vi "OBJ_parse_read_gear_data_response.vi"(8 "error_in":errorcluster, 11 "recordset_in":variant) -> (0 "error_out":errorcluster, 2 "Perform test?":bool)   [LabVIEW 2019]
uses:
  FGV/tristate_indicator_OBJ_test/FGV_tristate_indicator_OBJ_test.ctl
  FGV/test_button/FGV_OBJ_test_button.ctl
  <vilib>/addons/database/_DB Variant To Data/Database Variant To Data.xnode
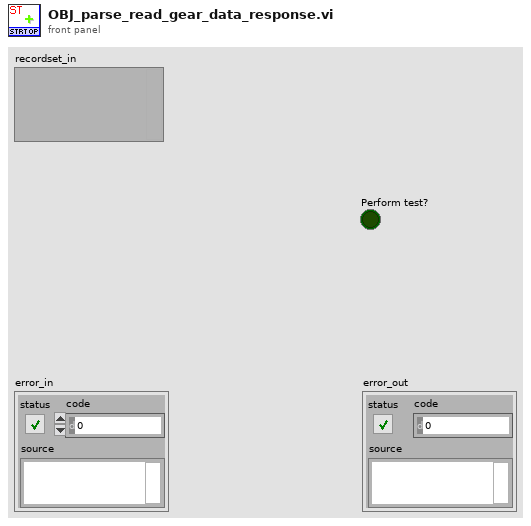
[diagram p1: front panel]
types:
  T1 = typedef "FGV_OBJ_test_button.ctl" = enum16{"initialize", "set_new_login", "set_message", "enable", "disable", "disable_gray", "translate"}
  T2 = typedef "FGV_tristate_indicator_OBJ_test.ctl" = enum16{"initialize", "ready", "pending", "OK", "NOK", "part_NOK", "routing_NOK", "repeat_NOK", "timeout", "translate", "error"}
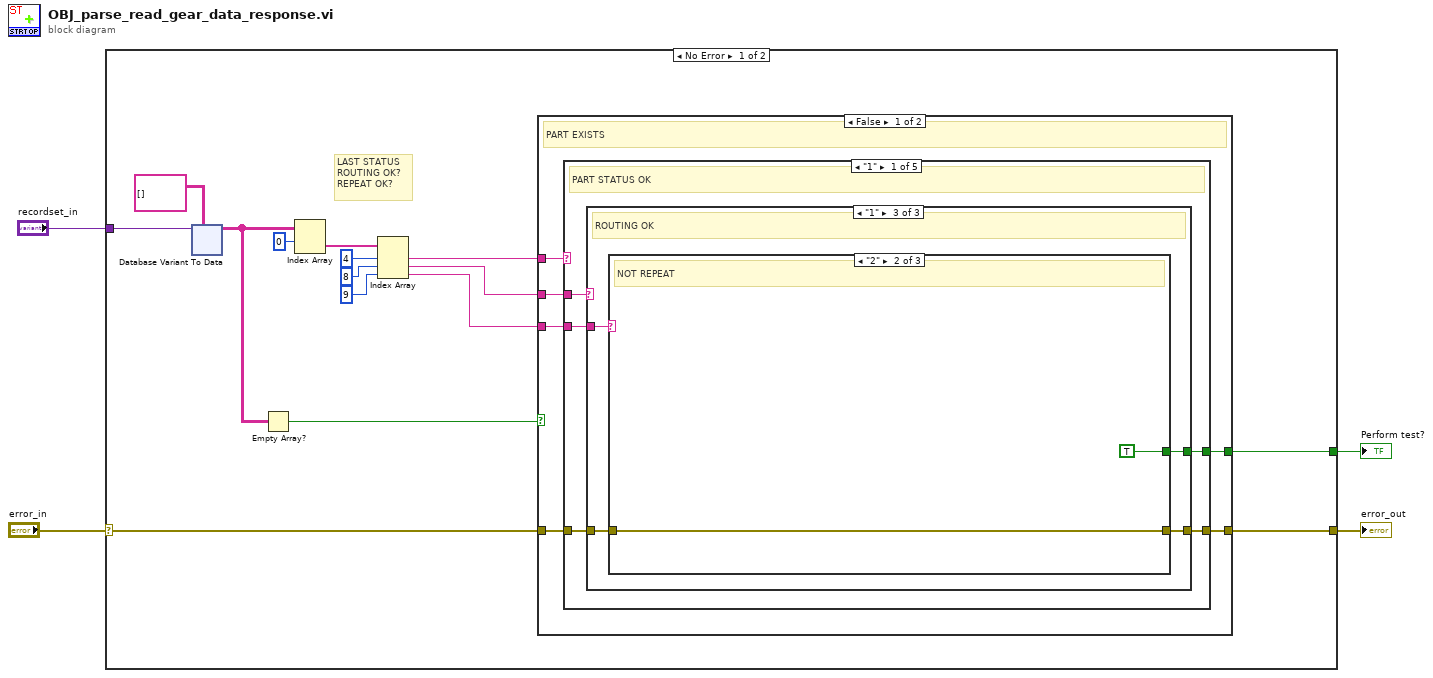
[diagram p0: block diagram]
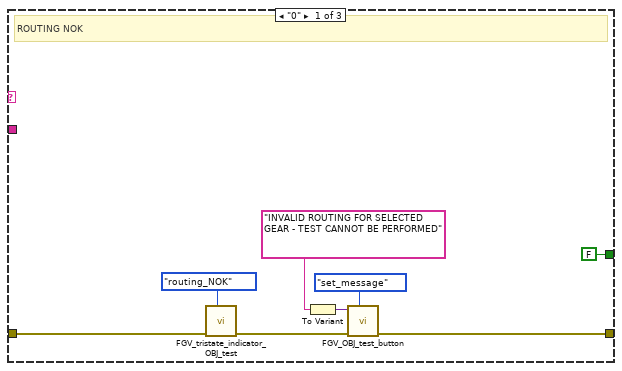
[diagram p2: hidden frame]
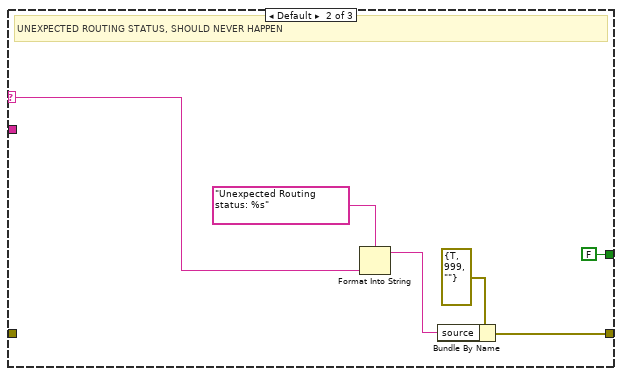
[diagram p3: hidden frame]
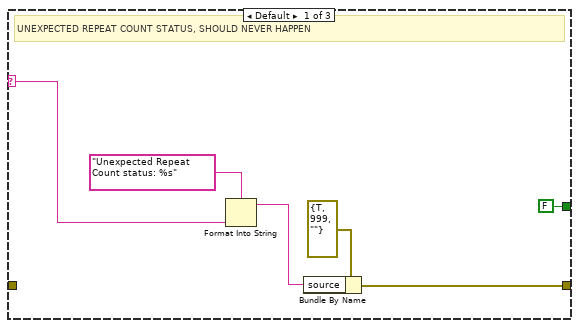
[diagram p4: hidden frame]
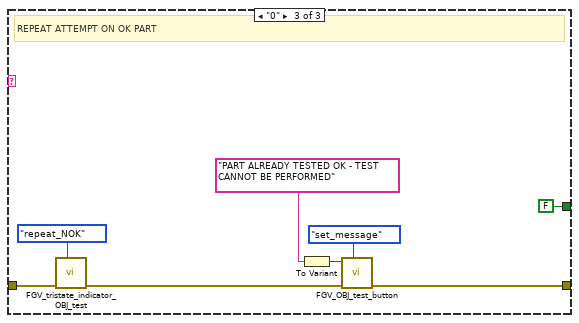
[diagram p5: hidden frame]
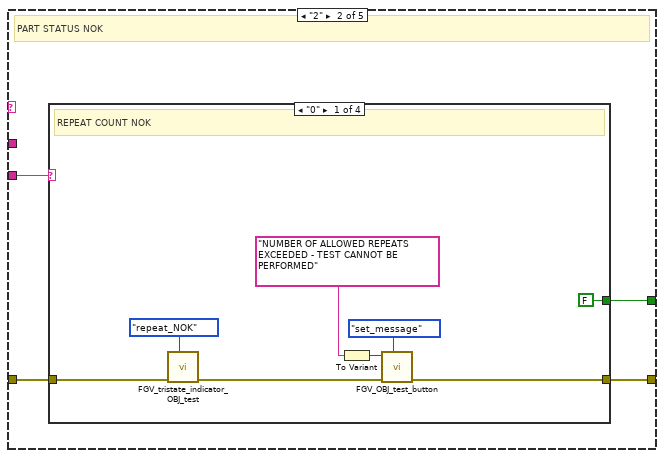
[diagram p6: hidden frame]
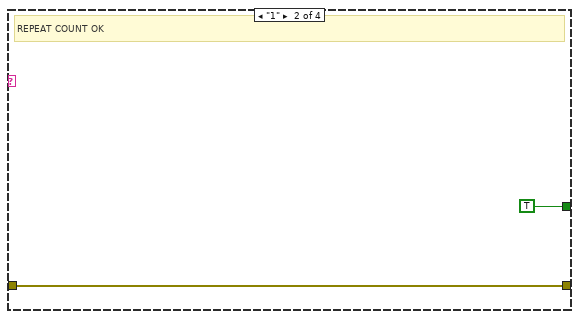
[diagram p7: hidden frame]
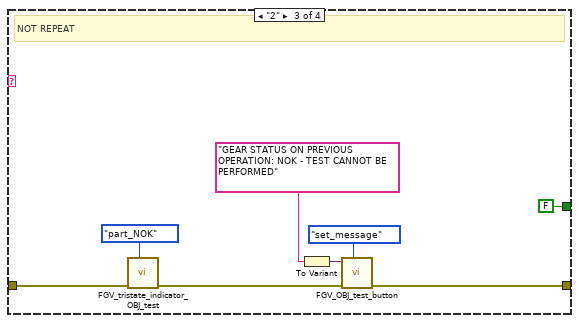
[diagram p8: hidden frame]
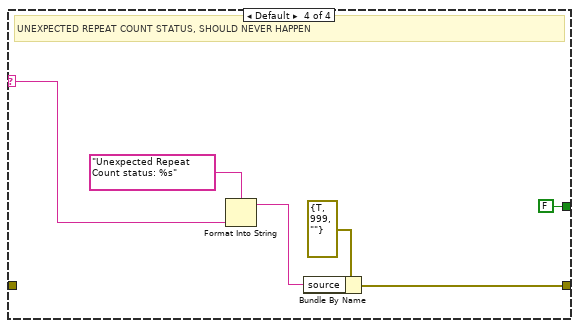
[diagram p9: hidden frame]
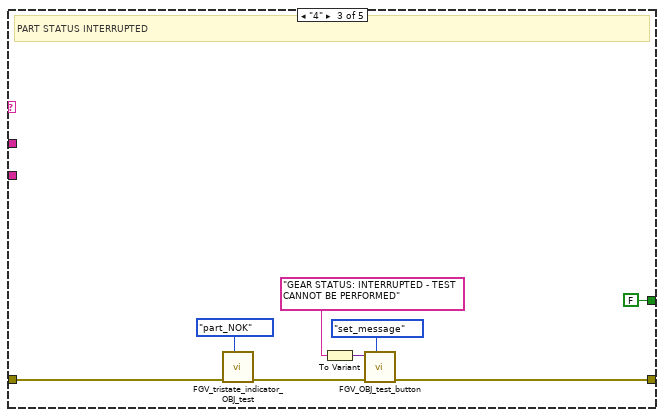
[diagram p10: hidden frame]
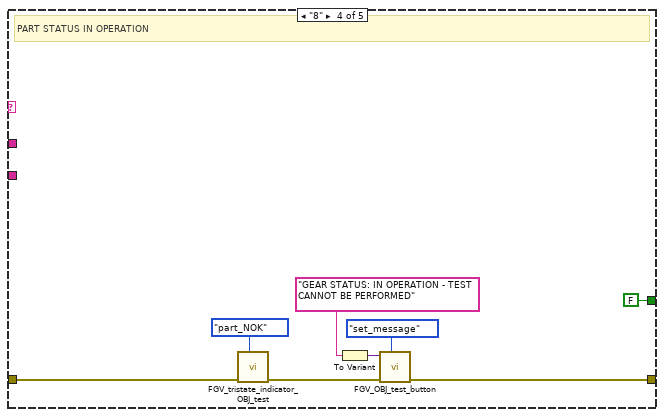
[diagram p11: hidden frame]
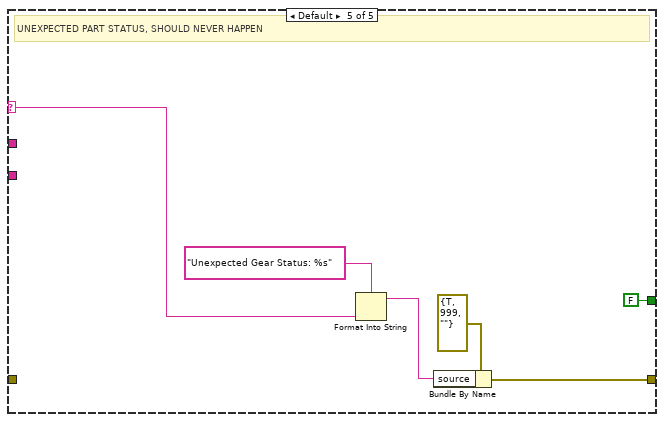
[diagram p12: hidden frame]
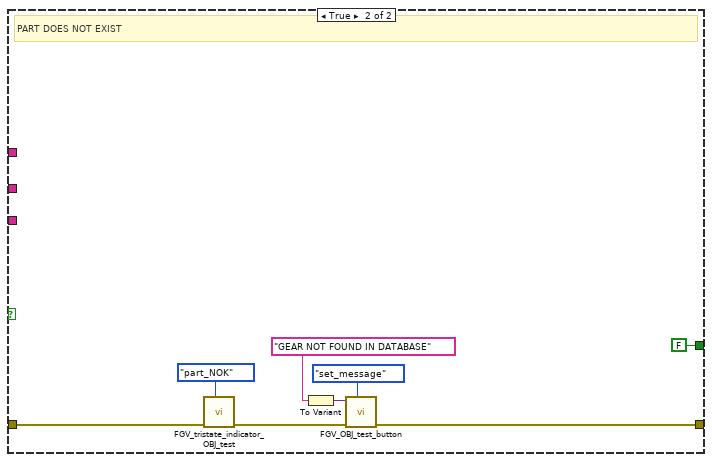
[diagram p13: hidden frame]
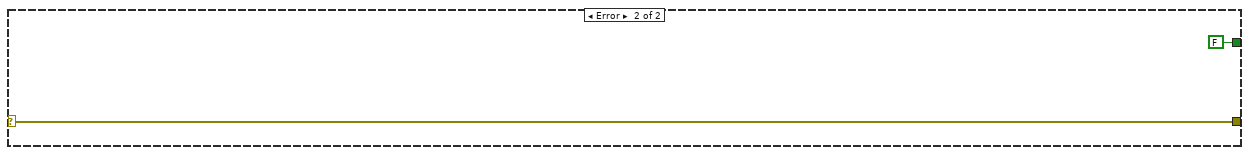
[diagram p14: hidden frame]
diagram:
  n1 = case shown="No Error" "error_in" {
    selector: "error_in" -> [w14 w156]
    tunnel: [w13 w156] -> w3
    tunnel: [w10 FALSE] -> w2
    tunnel: "recordset_in" -> [w9 _]
    frame No Error {
      # "LAST STATUS\nROUTING OK?\nREPEAT OK?"
      n2 = xnode "Database Variant To Data"("database variant"=w9, "type"=string[][] []) -> ("data"=w8:string[][])  [unwired: 1 in, 1 out]
      n3 = Empty Array?(array=w8) -> (empty?=w7:bool)
      n4 = Index Array(array=w8, index (row)=0) -> (element=w17:string[])  [unwired: 1 in]
      n5 = Index Array(array=w17, index #1=4 ("index"), index #2=8 ("index"), index #3=9 ("index")) -> (element #1=w15:string, element #2=w12:string, element #3=w11:string)
      n6 = case shown="False" w7 {
        tunnel: w15 -> [w57 _]
        tunnel: w14 -> [w56 w151]
        tunnel: [w55 w149] -> w13
        tunnel: w12 -> [w54 _]
        tunnel: w11 -> [w53 _]
        tunnel: [w52 FALSE] -> w10
        frame False {
          # "PART EXISTS"
          n7 = case shown="\"1\"" w57 {
            selector: w57 -> [_ _ _ _ w143]
            tunnel: w56 -> [w61 w100 w126 w134 _]
            tunnel: [w59 w99 w125 w133 w142] -> w55
            tunnel: w54 -> [w62 _ _ _ _]
            tunnel: w53 -> [w60 w97 _ _ _]
            tunnel: [w58 w98 FALSE FALSE FALSE] -> w52
            frame "1" {
              # "PART STATUS OK"
              n8 = case shown="\"1\"" w62 {
                selector: w62 -> [_ w72 _]
                tunnel: w61 -> [w64 _ w79]
                tunnel: w60 -> [_ _ w80]
                tunnel: [w63 w73 w78] -> w59
                tunnel: [FALSE FALSE w77] -> w58
                frame "0" {
                  # "ROUTING NOK"
                  n9 = call "FGV_tristate_indicator_OBJ_test.vi"("options"=FGV_tristate_indicator_OBJ_test."routing_NOK", "error_in"=w64) -> ("error_out"=w67:errorcluster)  [unwired: 9 in]
                  n10 = To Variant(anything="INVALID ROUTING FOR SELECTED GEAR - TEST CANNOT BE PERFORMED") -> (Variant=w66:variant)
                  n11 = call "FGV_OBJ_test_button.vi"("options"=FGV_OBJ_test_button."set_message", "error_in"=w67, "input"=w66) -> ("error_out"=w63:errorcluster)  [unwired: 8 in]
                }
                frame Default {
                  # "UNEXPECTED ROUTING STATUS, SHOULD NEVER HAPPEN"
                  n12 = Format Into String(format string="Unexpected Routing status: %s", w72) -> (resulting string=w74:string)  [unwired: 2 in, 1 out]
                  n13 = Bundle By Name(cluster=errorcluster {"status"=TRUE, "code"=999, "source"=""} ("error_in"), "source"=w74) -> (w73:errorcluster)
                }
                frame "1" {
                  # "ROUTING OK"
                  n14 = case shown="\"2\"" w80 {
                    selector: w80 -> [w82 _ _]
                    tunnel: w79 -> [_ w87 w90]
                    tunnel: [w85 w87 w89] -> w78
                    tunnel: [FALSE TRUE FALSE] -> w77
                    frame Default {
                      # "UNEXPECTED REPEAT COUNT STATUS, SHOULD NEVER HAPPEN"
                      n15 = Format Into String(format string="Unexpected Repeat Count status: %s", w82) -> (resulting string=w83:string)  [unwired: 2 in, 1 out]
                      n16 = Bundle By Name(cluster=errorcluster {"status"=TRUE, "code"=999, "source"=""} ("error_in"), "source"=w83) -> (w85:errorcluster)
                    }
                    frame "2" {
                      # "NOT REPEAT"
                    }
                    frame "0" {
                      # "REPEAT ATTEMPT ON OK PART"
                      n17 = call "FGV_tristate_indicator_OBJ_test.vi"("options"=FGV_tristate_indicator_OBJ_test."repeat_NOK", "error_in"=w90) -> ("error_out"=w93:errorcluster)  [unwired: 9 in]
                      n18 = To Variant(anything="PART ALREADY TESTED OK - TEST CANNOT BE PERFORMED") -> (Variant=w92:variant)
                      n19 = call "FGV_OBJ_test_button.vi"("options"=FGV_OBJ_test_button."set_message", "error_in"=w93, "input"=w92) -> ("error_out"=w89:errorcluster)  [unwired: 8 in]
                    }
                  }
                }
              }
            }
            frame "2" {
              # "PART STATUS NOK"
              n20 = case shown="\"0\"" w97 {
                selector: w97 -> [_ _ _ w120]
                tunnel: w100 -> [w102 w109 w112 _]
                tunnel: [w101 w109 w111 w123] -> w99
                tunnel: [FALSE TRUE FALSE FALSE] -> w98
                frame "0" {
                  # "REPEAT COUNT NOK"
                  n21 = call "FGV_tristate_indicator_OBJ_test.vi"("options"=FGV_tristate_indicator_OBJ_test."repeat_NOK", "error_in"=w102) -> ("error_out"=w105:errorcluster)  [unwired: 9 in]
                  n22 = To Variant(anything="NUMBER OF ALLOWED REPEATS EXCEEDED - TEST CANNOT BE PERFORMED") -> (Variant=w104:variant)
                  n23 = call "FGV_OBJ_test_button.vi"("options"=FGV_OBJ_test_button."set_message", "error_in"=w105, "input"=w104) -> ("error_out"=w101:errorcluster)  [unwired: 8 in]
                }
                frame "1" {
                  # "REPEAT COUNT OK"
                }
                frame "2" {
                  # "NOT REPEAT"
                  n24 = call "FGV_tristate_indicator_OBJ_test.vi"("options"=FGV_tristate_indicator_OBJ_test."part_NOK", "error_in"=w112) -> ("error_out"=w115:errorcluster)  [unwired: 9 in]
                  n25 = To Variant(anything="GEAR STATUS ON PREVIOUS OPERATION: NOK - TEST CANNOT BE PERFORMED") -> (Variant=w114:variant)
                  n26 = call "FGV_OBJ_test_button.vi"("options"=FGV_OBJ_test_button."set_message", "error_in"=w115, "input"=w114) -> ("error_out"=w111:errorcluster)  [unwired: 8 in]
                }
                frame Default {
                  # "UNEXPECTED REPEAT COUNT STATUS, SHOULD NEVER HAPPEN"
                  n27 = Format Into String(format string="Unexpected Repeat Count status: %s", w120) -> (resulting string=w121:string)  [unwired: 2 in, 1 out]
                  n28 = Bundle By Name(cluster=errorcluster {"status"=TRUE, "code"=999, "source"=""} ("error_in"), "source"=w121) -> (w123:errorcluster)
                }
              }
            }
            frame "4" {
              # "PART STATUS INTERRUPTED"
              n29 = call "FGV_tristate_indicator_OBJ_test.vi"("options"=FGV_tristate_indicator_OBJ_test."part_NOK", "error_in"=w126) -> ("error_out"=w129:errorcluster)  [unwired: 9 in]
              n30 = To Variant(anything="GEAR STATUS: INTERRUPTED - TEST CANNOT BE PERFORMED") -> (Variant=w128:variant)
              n31 = call "FGV_OBJ_test_button.vi"("options"=FGV_OBJ_test_button."set_message", "error_in"=w129, "input"=w128) -> ("error_out"=w125:errorcluster)  [unwired: 8 in]
            }
            frame "8" {
              # "PART STATUS IN OPERATION"
              n32 = call "FGV_tristate_indicator_OBJ_test.vi"("options"=FGV_tristate_indicator_OBJ_test."part_NOK", "error_in"=w134) -> ("error_out"=w137:errorcluster)  [unwired: 9 in]
              n33 = To Variant(anything="GEAR STATUS: IN OPERATION - TEST CANNOT BE PERFORMED") -> (Variant=w136:variant)
              n34 = call "FGV_OBJ_test_button.vi"("options"=FGV_OBJ_test_button."set_message", "error_in"=w137, "input"=w136) -> ("error_out"=w133:errorcluster)  [unwired: 8 in]
            }
            frame Default {
              # "UNEXPECTED PART STATUS, SHOULD NEVER HAPPEN"
              n35 = Format Into String(format string="Unexpected Gear Status: %s", w143) -> (resulting string=w144:string)  [unwired: 2 in, 1 out]
              n36 = Bundle By Name(cluster=errorcluster {"status"=TRUE, "code"=999, "source"=""} ("error_in"), "source"=w144) -> (w142:errorcluster)
            }
          }
        }
        frame True {
          # "PART DOES NOT EXIST"
          n37 = call "FGV_tristate_indicator_OBJ_test.vi"("options"=FGV_tristate_indicator_OBJ_test."part_NOK", "error_in"=w151) -> ("error_out"=w150:errorcluster)  [unwired: 9 in]
          n38 = To Variant(anything="GEAR NOT FOUND IN DATABASE") -> (Variant=w148:variant)
          n39 = call "FGV_OBJ_test_button.vi"("options"=FGV_OBJ_test_button."set_message", "error_in"=w150, "input"=w148) -> ("error_out"=w149:errorcluster)  [unwired: 8 in]
        }
      }
    }
    frame Error {
    }
  }
  "error_out" <- w3
  "Perform test?" <- w2
